vi "Tosca-Init AI Plot Properties.vi"(0 "which kind":string, 5 "graph":refnum<vi>, 7 "names":string[](array[string]), 9 "first color":i32, 11 "error in (no error)":errorcluster) -> (8 "map":T1[](array[typedef]), 10 "next color":i32, 15 "error out":errorcluster)   [LabVIEW 2020]
uses:
  Typedefs/Tosca-AI Plot Properties.ctl
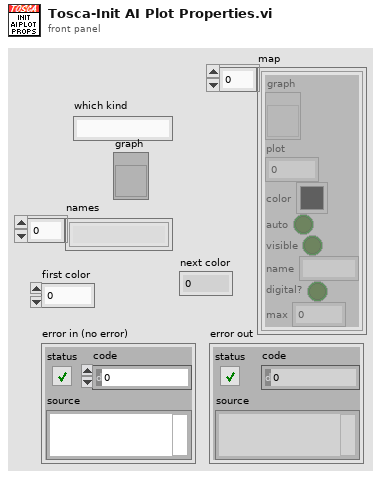
[diagram p1: front panel]
types:
  T1 = typedef "Tosca-AI Plot Properties.ctl" = cluster{"graph":refnum<vi>, "plot":i32, "color":u32, "auto":bool, "visible":bool, "name":string, "digital?":bool, "max":dbl}
  T2 = cluster{"color":u32, "visible":bool, "auto":bool, "max":dbl}
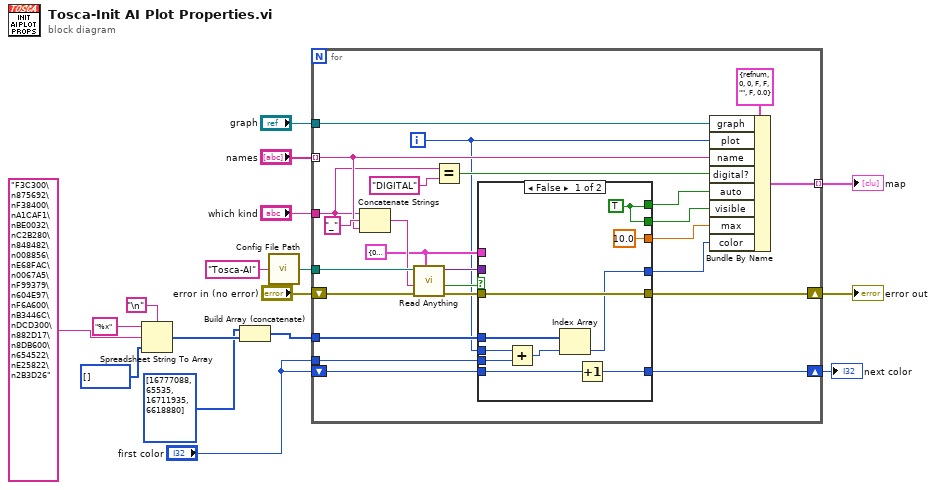
[diagram p0: block diagram]
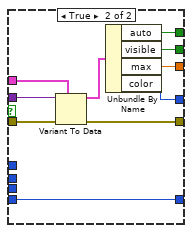
[diagram p2: hidden frame]
diagram:
  n1 = Spreadsheet String To Array(delimiter (Tab)="\n", format string="%x", spreadsheet string="F3C300\n875692\nF38400\nA1CAF1\nBE0032\nC2B280\n848482\n008856\nE68FAC\n0067A5\nF99379\n604E97\nF6A600\nB3446C\nDCD300\n882D17\n8DB600\n654522\nE25822\n2B3D26", array type (2D Dbl)=u32[] []) -> (array=w5:u32[])
  n2 = Build Array (concatenate)(u32[] [16777088, 65535, 16711935, 6618880], w5) -> (w4:u32[])
  n3 = call "Config File Path.vi"("AppName"="Tosca-AI") -> ("Default config file name"=w12:path)
  n4 = for {
    tunnel: "graph" -> [w41]
    tunnel: "names" -> [w38] mode=indexing
    tunnel: [w40] -> w14 mode=indexing
    tunnel: "which kind" -> [w23]
    tunnel: w12 -> [w37]
    shift-right: [w30] -> w10
    shift-left: "error in (no error)" -> [w33]
    shift-right: [w25] -> w2
    shift-left: "first color" -> [w26]
    tunnel: w4 -> [w24]
    tunnel: "first color" -> [w18]
    i -> [w19]
    w31 = T2 {"color"=0, "visible"=FALSE, "auto"=FALSE, "max"=0.0}
    n5 = Concatenate Strings(w23, "_" ("string"), w38) -> (w36:string)
    n6 = call "Read Anything.vi"("Type of Anything"=w31, "Error In"=w33, "Section Name (Name of \"Type of Anything\")"=w36, "Path (dialog)"=w37) -> ("Error Out"=w35:errorcluster, "Found?"=w34:bool, "Anything"=w32:variant)  [unwired: 5 in]
    n7 = Equal?(x=w23, y="DIGITAL" ("x")) -> (x = y?=w21:bool)
    n8 = case shown="False" w34 {
      tunnel: w35 -> [w52 w62]
      tunnel: w32 -> [_ w60]
      tunnel: w31 -> [_ w61]
      tunnel: [w52 w59] -> w30
      tunnel: [w51 w57] -> w29
      tunnel: [w51 w56] -> w28
      tunnel: [w47 w55] -> w27
      tunnel: w26 -> [w48 w54]
      tunnel: [w50 w54] -> w25
      tunnel: w24 -> [w49 _]
      tunnel: [10.0 ("max") w53] -> w20
      tunnel: w19 -> [w45 _]
      tunnel: w18 -> [w43 _]
      frame False {
        w51 = TRUE ("auto")
        n9 = Add(x=w45, y=w43) -> (x+y=w44:i32)
        n10 = Index Array(array=w49, index=w44) -> (element=w47:u32)
        n11 = Increment(x=w48) -> (x+1=w50:i32)
      }
      frame True {
        n12 = Variant To Data(error in=w62, type=w61, Variant=w60) -> (data=w58:T2, error out=w59:errorcluster)
        n13 = Unbundle By Name(w58) -> ("auto"=w57:bool, "visible"=w56:bool, "max"=w53:dbl, "color"=w55:u32)
      }
    }
    n14 = Bundle By Name(cluster=T1 {"graph"=refnum, "plot"=0, "color"=0, "auto"=FALSE, "visible"=FALSE, "name"="", "digital?"=FALSE, "max"=0.0}, "graph"=w41, "plot"=w19, "name"=w38, "digital?"=w21, "auto"=w29, "visible"=w28, "max"=w20, "color"=w27) -> (w40:T1)
  }
  "error out" <- w10
  "map" <- w14
  "next color" <- w2
